vi "Configure User Defined Function.vi"(5 "Function Number (1)":i32=1 min=1 max=20 step=1, 7 "Enable User Defined Function (T: Enable)":bool=TRUE, 8 "error in (no error)":errorcluster, 10 "Expression (Empty)":string, 11 "VISA resource name":refnum<visa-resource-name>) -> (0 "error out":errorcluster, 3 "VISA resource name out":refnum<visa-resource-name>)   [LabVIEW 2021, in "Yokogawa WT1800 Series.lvlib"]
doc: "Combine function symbols to create equations and use the numeric data of the combined functions to determine the value of the equation."
uses:
  <instrlib>/Yokogawa WT1800 Series/Yokogawa WT1800 Series.lvlib
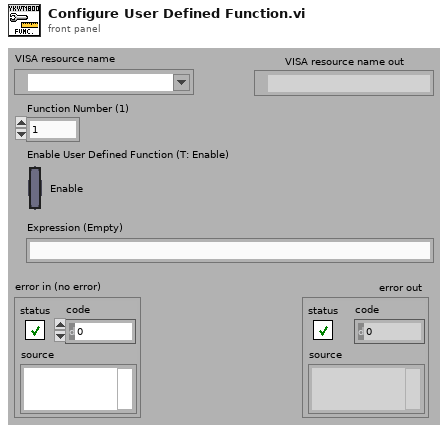
[diagram p1: front panel]
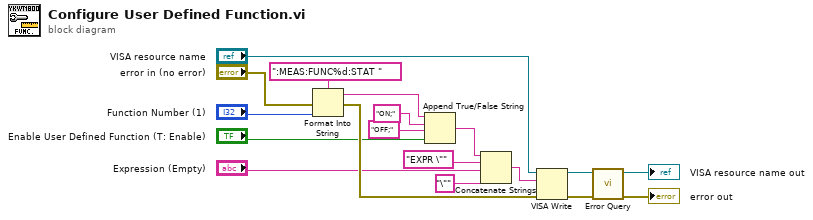
[diagram p0: block diagram]
diagram:
  n1 = Format Into String(format string=":MEAS:FUNC%d:STAT " ("形式文字列"), error in="error in (no error)", "Function Number (1)") -> (resulting string=w8:string, error out=w12:errorcluster)  [unwired: 1 in]
  n2 = Append True/False String ("True/False 文字列を追加")(1:"Enable User Defined Function (T: Enable)", 2:"OFF;", 3:"ON;", 4:w8) -> (0:w5:string)
  n3 = Concatenate Strings(w5, "EXPR \"" ("文字列"), "Expression (Empty)", "\"" ("文字列")) -> (w3:string)
  n4 = VISA Write ("VISA書き込み")(VISA resource name="VISA resource name", write buffer=w3, error in (no error)=w12) -> (VISA resource name out=w18:refnum<visa-resource-name>, error out=w17:errorcluster)  [unwired: 1 out]
  n5 = call <instrlib>:"Error Query.vi"("error in (no error)"=w17, "VISA resource name"=w18) -> ("error out"=→"error out":errorcluster, "VISA resource name out"=→"VISA resource name out":refnum<visa-resource-name>)  [unwired: 6 in, 2 out]
